vi "MakeFolderIfNeed.vi"(11 "folder path":path) -> (3 "dup folder path":path)   [LabVIEW 2013]
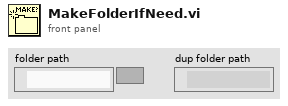
[diagram p1: front panel]
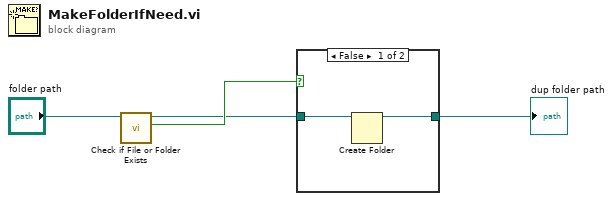
[diagram p0: block diagram]
diagram:
  n1 = call <vilib>:"Check if File or Folder Exists.vi"("path"="folder path") -> ("file or folder exists?"=w3:bool, "dup path"=w2:path)  [unwired: 8 in, 1 out]
  n2 = case shown="False" w3 {
    tunnel: [w6 w7] -> w1
    tunnel: w2 -> [w5 w7]
    frame False {
      n3 = Create Folder(path (use dialog)=w5) -> (created path=w6:path)  [unwired: 2 in, 2 out]
    }
    frame True {
    }
  }
  "dup folder path" <- w1
